vi "64 RMS.vi"() -> ()   [LabVIEW 2017]
uses:
  <vilib>/Analysis/baseanly.llb/Mean (DBL).vi
  <vilib>/Analysis/NI_AALBase.lvlib
panel:
  out "TDC 32 Width":dbl[](graph)=[-0.6783163457252961, 34.80339865309444, -9.301868316936371, -18.575029046661424, -30.46824115548442, -36.068889974290876, -48.12167844719457, -62.45045124910451, -82.61219931936799, -67.52504545488544, -82.18213797919361, -74.58060582693615, -82.56997925436134, -51.89278804838313, -74.89460611630447, -18.140506580336282, -54.34241861431395, 120.78238637788458, 104.77997514317252, 69.37552504098075, 102.67355117145733, 61.80624599007051, 69.19828291963655, 56.38383575637289, 65.54038193174377, 81.65259235989721, 59.02039418272081, 52.81620434909051, 72.46570862393186, 17.962024313646307, 60.3235058067138, 51.75675031672855, 56.5848106452265, 45.431151381143735, 48.336679201226005, 10.391614557583782, 32.39305706018139, -12.86505630083905, -24.22287886989784, -15.211095332141797, -12.471040103140627, -7.020617140658874, -16.741559776427525, -21.080385174466098, -1.214389654830226, -36.76592185679817, -45.26070308895697, 15.57295580171187, -33.053175507633306, -37.140407160289904, -62.42416008241627, -12103.8678050851, -12121.48251904026, -12111.404616944672, -12129.543609930342, -12139.843547353412, -12129.977664947211, -12131.654983175655, -12134.08824321654, -12113.99974215647, -12112.278518000594, -12102.802796490787, -12126.243066943878]
  in  "PMT Num Channel":i32=64
  out "TDC 32 Pre RMS 2":dbl[](graph)
  out "TDC 32 Mean 2":dbl[](graph)=[0.0, -135.09479077989525, -421.8271505306632, -840.8446778298572, -1162.0976991710277, -1612.7332666304121, -2198.59017285921, -2560.663067796938, -2635.055025403253, -2231.1708563380016, -2195.002950279124, -1580.3730444661662, -1326.1414516725524, -1107.6882588350188, -612.4428634104521, -418.3344995069555, -181.55837998871735, -553.1504945996667, -839.4835673473254, -924.4151651207177, -1354.6877899459462, -1876.633411331489, -2226.4242092546738, -2150.03492136841, -1877.2355072689136, -1778.347255928683, -1323.9390592383058, -710.8504740240475, -576.8078492540101, -276.2199801150382, 188.3439838906523, 324.0294182912872]
  in  "Width大于信号周期":dbl=10000.0
  in  "Width小于信号周期":dbl=10000000.0
  in  "Post大于信号周期":dbl
  in  "Post小于信号周期":dbl=25000.0
  in  "Pre大于信号周期":dbl
  in  "Pre小于信号周期":dbl=25500.0
  in  "min bin 3":i32=30
  in  "length 3":dbl=60.0 format="%#_13g"
  out "Fitting RMS 2":dbl=7.681145747868608
  out "Array 3":dbl[](array[numeric])=[0.0, 4.475261371081126, 3.162544268461357, 2.924189728577925, 4.462904629576637, 4.688451182126854, 4.149795436251731, 5.294255584605741, 4.358239562408714, 5.964552050869855, 6.274622613679179, 4.820259051506523, 6.210237569711836, 6.202576111524344, 5.12191356026047, 5.902693786358635, 7.264783281499365, 3.8782644204457255, 6.15892371349985, 5.6565100281603495, 5.6445556358933535, 5.586306730858833, 5.237143591840878, 7.583770998832869, 5.692958951594319, 4.962442273104816, 5.385209825663387, 6.281457453209248, 4.513090750771602, 4.263987705812667, 4.44121495773946, 4.025581062368119]
  out "index 3":i32
  out "Fitting RMS":dbl=3.2734913936560712
  in  "String":string
  out "cal 3":cluster{"cal 2":dbl[]}[](graph)=[{"cal 2"=[0.0, 4.114652313560727, 4.4615536591768565, 4.487541869293653, 4.305805863389491, 4.3919731471213845, 4.293945065128187, 3.9563450305643455, 4.781590920128164, 4.566725321246964, 3.769905678360813, 3.996457081541512, 3.6292687673693096, 4.6661813542211945, 3.9547291663385615, 4.0878496237189195, 5.193601946935443, 4.363571307074085, 4.620812080547306, 4.68636099579301, 4.522595786195377, 4.94953151612554, 4.20504962269455, 4.5858390402275155, 4.63399159695198, 5.369311213376012, 4.839189336674422, 5.220406472025208, 4.474735648398492, 4.088850343918244, 5.168763522181636, 6.520882565694521]}, {"cal 2"=[0.0, 4.475261371081126, 3.162544268461357, 2.924189728577925, 4.462904629576637, 4.688451182126854, 4.149795436251731, 5.294255584605741, 4.358239562408714, 5.964552050869855, 6.274622613679179, 4.820259051506523, 6.210237569711836, 6.202576111524344, 5.12191356026047, 5.902693786358635, 7.264783281499365, 3.8782644204457255, 6.15892371349985, 5.6565100281603495, 5.6445556358933535, 5.586306730858833, 5.237143591840878, 7.583770998832869, 5.692958951594319, 4.962442273104816, 5.385209825663387, 6.281457453209248, 4.513090750771602, 4.263987705812667, 4.44121495773946, 4.025581062368119]}]
  out "post mean":dbl=3.154553539854668 format="%0.2f"
  out "pre mean":dbl=2.9457244798960076 format="%0.2f"
  out "mean":dbl=3.050139009875338 format="%0.2f"
  out "TDC 32 Mean":dbl[](graph)=[0.0, -36.996434242557854, -31.313627065973662, -21.077383139604187, 2.6241265645144156, 24.179747631180753, 2.7343041360305027, -30.431283162442877, 18.929146350224407, 35.626740082844826, 54.916933857204114, 38.31421986338976, 51.65477997851549, 14.6334264613231, 63.72841817768095, 23.989321006770542, 66.44079691895976, -2.810644526473722, -130.76823833968274, -83.04624565073621, -125.70406933559532, -120.26787383317914, -78.81175803979941, -76.26600047186471, -124.72740831159858, -86.923123129569, -112.60533075805586, -80.56440015739442, -93.43063512184393, -101.85614274031633, -58.36081718509212, -71.76328499120083, -110.40069925774178, -83.1465185905702, -45.32711285598063, -52.80271804532156, -12.349259962253637, -6.78472000965643, 19.69497358721831, -2.6869885934701703, -0.49182237994686606, 30.518656522275663, 22.293804071974055, 12.59663288956947, 6.842670087488456, -17.05003568301032, -5.350597835875373, 17.811916976727968, 3.882015796675974, 36.65946347529074, 6.0177148567894845, 50.32927610106109, 12120.695864120817, 12102.81226011086, 12106.473027754682, 12166.901296162248, 12132.2829669936, 12127.91935865152, 12112.96936554167, 12147.343894796079, 12110.6243252432, 12131.056590850796, 12139.238157468637, 12131.590924217124]
  out "cal 2":cluster{"cal 2":dbl[]}[](graph)=[{"cal 2"=[0.0, 2.7660591431756636, 2.7965204008011693, 2.8371751476759077, 2.9687865748397413, 2.586901217982678, 3.049603258650606, 2.7769429000377315, 2.84337439739946, 2.8079919817042938, 3.0911315648646758, 3.2064489186545337, 2.899310886145602, 3.307008327270206, 2.90831028930621, 3.418607736993944, 2.991778379065165, 3.1044560328618847, 2.8635383951772084, 2.874130589680789, 2.9022368004793555, 3.163327380796549, 3.095057673087491, 3.017902652759673, 2.576954383186888, 2.830253201212209, 3.0679451279799497, 3.0082959014666697, 3.0310317195983947, 3.086400717933539, 3.148829226197087, 2.9710914995519375, 3.1027831871783977, 3.081309500479302, 3.0130135668078113, 3.129637095585219, 3.027166346566586, 2.9275365165118745, 2.856538471442075, 2.802569477786886, 3.0221181838965676, 3.0701711249384998, 3.123228137730836, 3.091689538434885, 2.9169499835656345, 3.2171659335383005, 2.9161334166545054, 3.156954195781715, 3.4267992870209865, 2.763287658090245, 2.9777255480248073, 2.9171925704161987, 2.966870830785901, 2.8776645339995643, 2.60596569982052, 3.0716380760397723, 3.017306157019706, 3.004246243333819, 3.0730206629174335, 3.037578499717302, 3.078007168642431, 2.952557438808163, 3.1355522957812796, 3.168586939490012]}, {"cal 2"=[0.0, 2.8996020427561886, 2.9895727123516944, 3.063090569150334, 2.885454310411448, 3.308199160492238, 2.8929806886235356, 3.1201842138819305, 2.7175292754088933, 3.2853680454446224, 3.4020354438142792, 3.4286914898543315, 3.276135144500932, 3.36085761963916, 3.2767937308862245, 3.4073773280141952, 3.2097845553822832, 3.124423833048686, 3.1124194853662472, 3.201558278093965, 3.025530124534342, 2.9839245800581313, 3.1800101711476065, 2.955793860682045, 3.2429221091245233, 2.9937445582570916, 2.9432208257186643, 3.149619864411783, 3.2718821210784856, 3.5334178494461552, 3.4373358702503625, 3.3677472097516246, 3.6041042638956777, 3.4388784451735224, 3.4801093500010754, 3.046059251257246, 3.2320592552775222, 3.193104588644505, 3.352133295854613, 3.5929937145986566, 3.1733456599894576, 3.1702333717532403, 3.1843260581136894, 3.1915311308326313, 2.990203209342016, 3.111223016994537, 3.2063459292445002, 3.3140730928092825, 3.406148065853031, 3.46159765385004, 3.3981654931647975, 3.162194273391769, 3.275580228314425, 3.1277255614951605, 3.0185159184215657, 3.078378013806016, 3.0340271987123693, 3.172771154107615, 3.4402058505393294, 3.1092898332858816, 3.2674772912638206, 3.1359517649189352, 3.201976150553741, 3.2734913936560712]}]
  in  "min bin 2":i32=30
  in  "length 2":dbl=60.0 format="%#_13g"
  out "Array 2":dbl[](array[numeric])=[0.0, 2.8996020427561886, 2.9895727123516944, 3.063090569150334, 2.885454310411448, 3.308199160492238, 2.8929806886235356, 3.1201842138819305, 2.7175292754088933, 3.2853680454446224, 3.4020354438142792, 3.4286914898543315, 3.276135144500932, 3.36085761963916, 3.2767937308862245, 3.4073773280141952, 3.2097845553822832, 3.124423833048686, 3.1124194853662472, 3.201558278093965, 3.025530124534342, 2.9839245800581313, 3.1800101711476065, 2.955793860682045, 3.2429221091245233, 2.9937445582570916, 2.9432208257186643, 3.149619864411783, 3.2718821210784856, 3.5334178494461552, 3.4373358702503625, 3.3677472097516246, 3.6041042638956777, 3.4388784451735224, 3.4801093500010754, 3.046059251257246, 3.2320592552775222, 3.193104588644505, 3.352133295854613, 3.5929937145986566, 3.1733456599894576, 3.1702333717532403, 3.1843260581136894, 3.1915311308326313, 2.990203209342016, 3.111223016994537, 3.2063459292445002, 3.3140730928092825, 3.406148065853031, 3.46159765385004, 3.3981654931647975, 3.162194273391769, 3.275580228314425, 3.1277255614951605, 3.0185159184215657, 3.078378013806016, 3.0340271987123693, 3.172771154107615, 3.4402058505393294, 3.1092898332858816, 3.2674772912638206, 3.1359517649189352, 3.201976150553741, 3.2734913936560712]
  out "TOT":dbl[](graph)=[0.0, 2.8996020427561886, 2.9895727123516944, 3.063090569150334, 2.885454310411448, 3.308199160492238, 2.8929806886235356, 3.1201842138819305, 2.7175292754088933, 3.2853680454446224, 3.4020354438142792, 3.4286914898543315, 3.276135144500932, 3.36085761963916, 3.2767937308862245, 3.4073773280141952, 3.2097845553822832, 3.124423833048686, 3.1124194853662472, 3.201558278093965, 3.025530124534342, 2.9839245800581313, 3.1800101711476065, 2.955793860682045, 3.2429221091245233, 2.9937445582570916, 2.9432208257186643, 3.149619864411783, 3.2718821210784856, 3.5334178494461552, 3.4373358702503625, 3.3677472097516246, 3.6041042638956777, 3.4388784451735224, 3.4801093500010754, 3.046059251257246, 3.2320592552775222, 3.193104588644505, 3.352133295854613, 3.5929937145986566, 3.1733456599894576, 3.1702333717532403, 3.1843260581136894, 3.1915311308326313, 2.990203209342016, 3.111223016994537, 3.2063459292445002, 3.3140730928092825, 3.406148065853031, 3.46159765385004, 3.3981654931647975, 3.162194273391769, 3.275580228314425, 3.1277255614951605, 3.0185159184215657, 3.078378013806016, 3.0340271987123693, 3.172771154107615, 3.4402058505393294, 3.1092898332858816, 3.2674772912638206, 3.1359517649189352, 3.201976150553741, 3.2734913936560712]
  out "index 2":i32=126
  in  "length":dbl=200.0 format="%#_13g"
  in  "min bin":i32=100
  out "index":i32=126
  out "TOA":dbl[](graph)=[0.0, 2.7660591431756636, 2.7965204008011693, 2.8371751476759077, 2.9687865748397413, 2.586901217982678, 3.049603258650606, 2.7769429000377315, 2.84337439739946, 2.8079919817042938, 3.0911315648646758, 3.2064489186545337, 2.899310886145602, 3.307008327270206, 2.90831028930621, 3.418607736993944, 2.991778379065165, 3.1044560328618847, 2.8635383951772084, 2.874130589680789, 2.9022368004793555, 3.163327380796549, 3.095057673087491, 3.017902652759673, 2.576954383186888, 2.830253201212209, 3.0679451279799497, 3.0082959014666697, 3.0310317195983947, 3.086400717933539, 3.148829226197087, 2.9710914995519375, 3.1027831871783977, 3.081309500479302, 3.0130135668078113, 3.129637095585219, 3.027166346566586, 2.9275365165118745, 2.856538471442075, 2.802569477786886, 3.0221181838965676, 3.0701711249384998, 3.123228137730836, 3.091689538434885, 2.9169499835656345, 3.2171659335383005, 2.9161334166545054, 3.156954195781715, 3.4267992870209865, 2.763287658090245, 2.9777255480248073, 2.9171925704161987, 2.966870830785901, 2.8776645339995643, 2.60596569982052, 3.0716380760397723, 3.017306157019706, 3.004246243333819, 3.0730206629174335, 3.037578499717302, 3.078007168642431, 2.952557438808163, 3.1355522957812796, 3.168586939490012]
  out "Array":dbl[](array[numeric])=[0.0, 2.7660591431756636, 2.7965204008011693, 2.8371751476759077, 2.9687865748397413, 2.586901217982678, 3.049603258650606, 2.7769429000377315, 2.84337439739946, 2.8079919817042938, 3.0911315648646758, 3.2064489186545337, 2.899310886145602, 3.307008327270206, 2.90831028930621, 3.418607736993944, 2.991778379065165, 3.1044560328618847, 2.8635383951772084, 2.874130589680789, 2.9022368004793555, 3.163327380796549, 3.095057673087491, 3.017902652759673, 2.576954383186888, 2.830253201212209, 3.0679451279799497, 3.0082959014666697, 3.0310317195983947, 3.086400717933539, 3.148829226197087, 2.9710914995519375, 3.1027831871783977, 3.081309500479302, 3.0130135668078113, 3.129637095585219, 3.027166346566586, 2.9275365165118745, 2.856538471442075, 2.802569477786886, 3.0221181838965676, 3.0701711249384998, 3.123228137730836, 3.091689538434885, 2.9169499835656345, 3.2171659335383005, 2.9161334166545054, 3.156954195781715, 3.4267992870209865, 2.763287658090245, 2.9777255480248073, 2.9171925704161987, 2.966870830785901, 2.8776645339995643, 2.60596569982052, 3.0716380760397723, 3.017306157019706, 3.004246243333819, 3.0730206629174335, 3.037578499717302, 3.078007168642431, 2.952557438808163, 3.1355522957812796, 3.168586939490012]
  in  "base channel":i32
  in  "file path (dialog if empty)":path=path "G:/tdc/2017/data/test_20250326_071915.csv"
  # "G:\\tdc\\2017\\test_20230328_085653.csv"
  # "G:\\tdc\\2017\\test_20230905_020448.csv   2.8 ps"
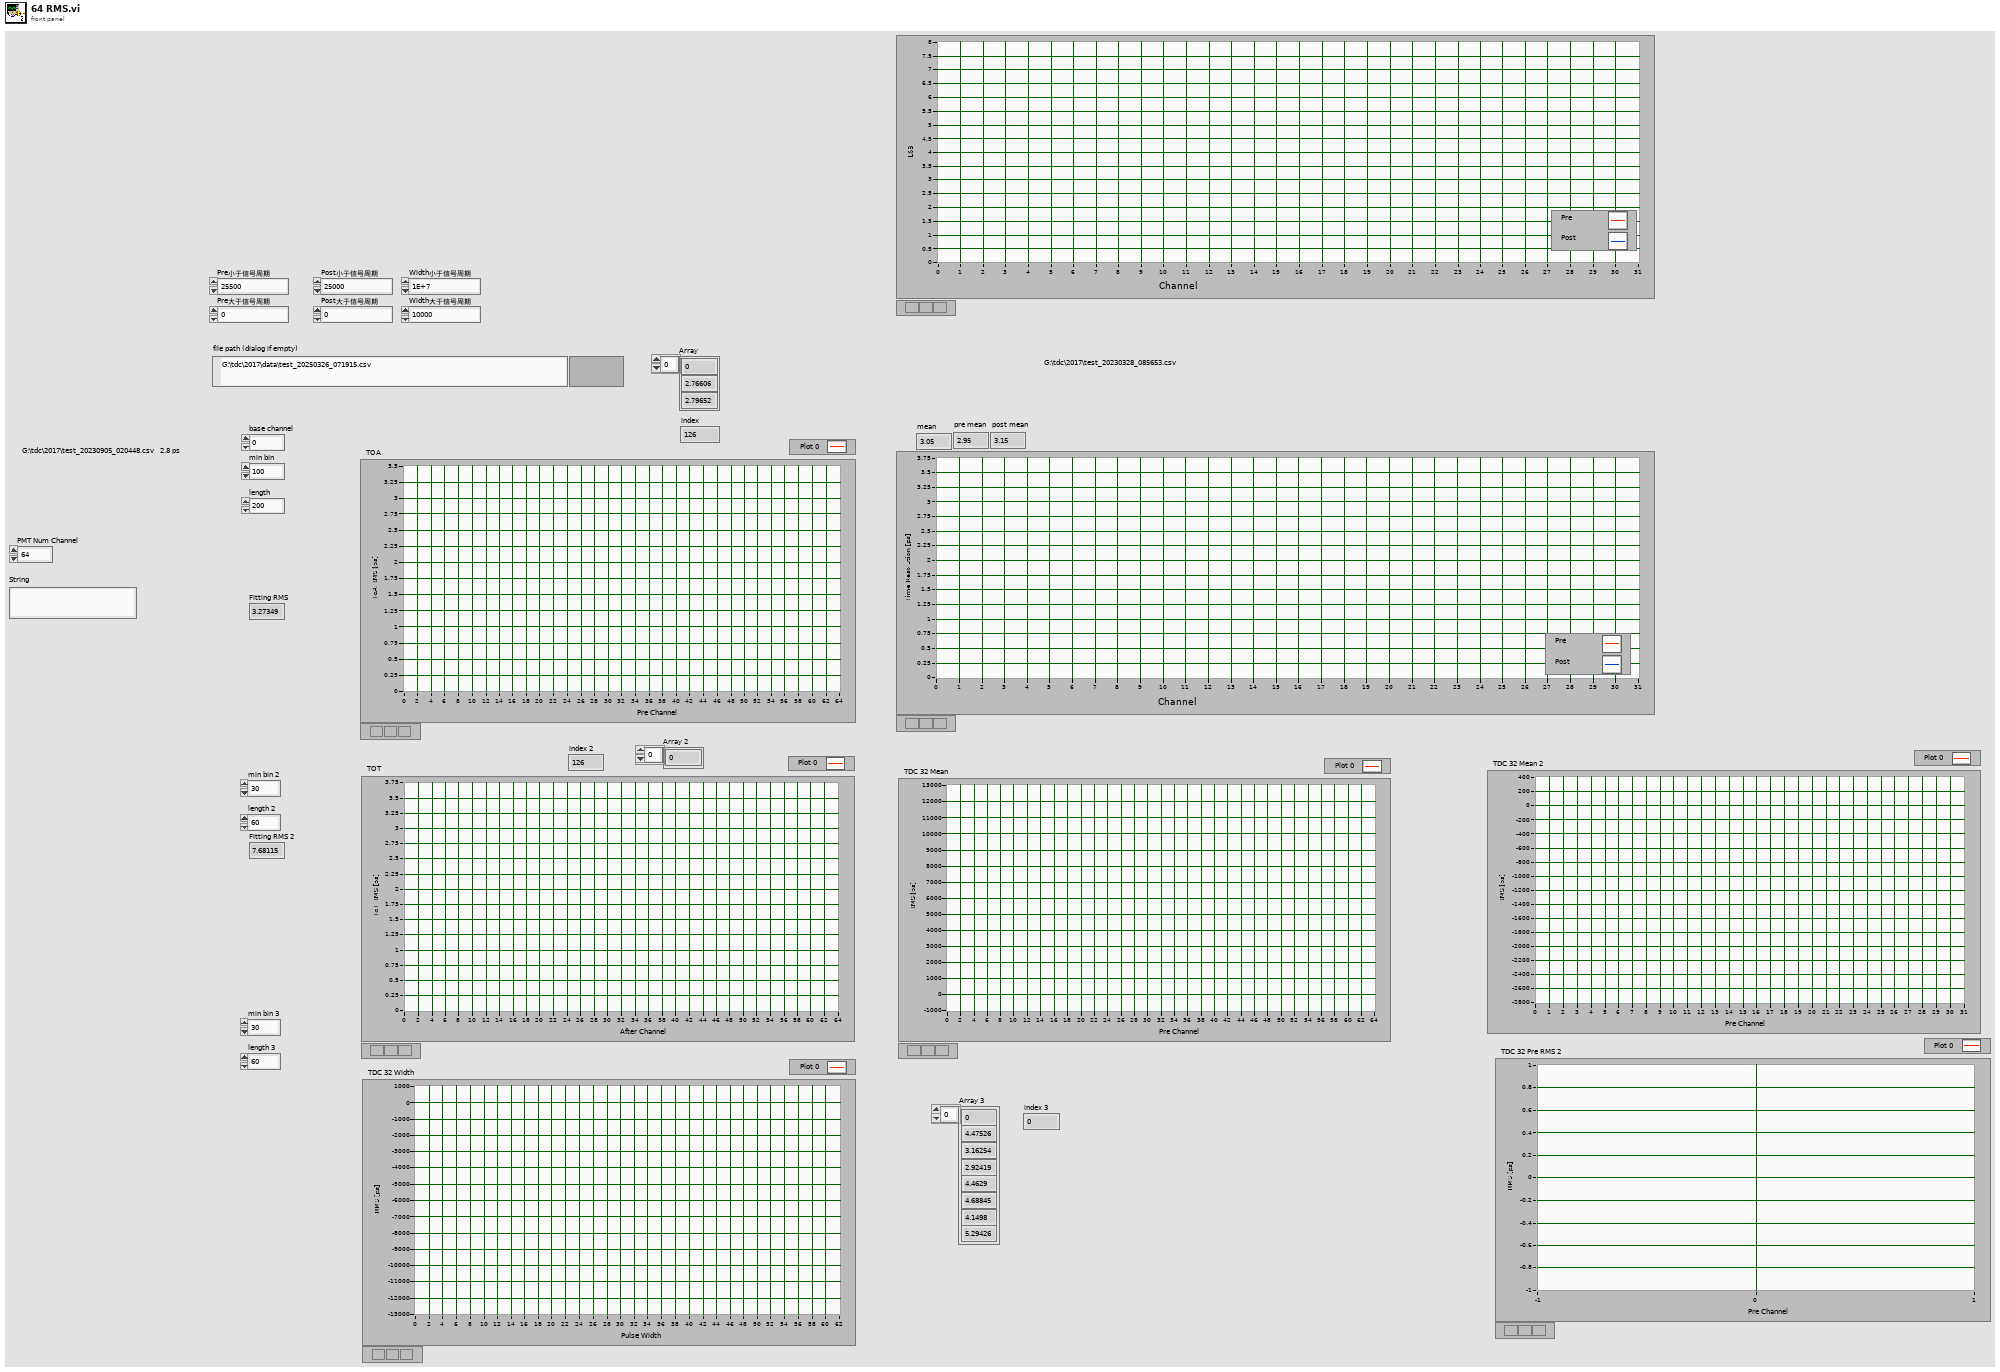
[diagram p1: front panel]
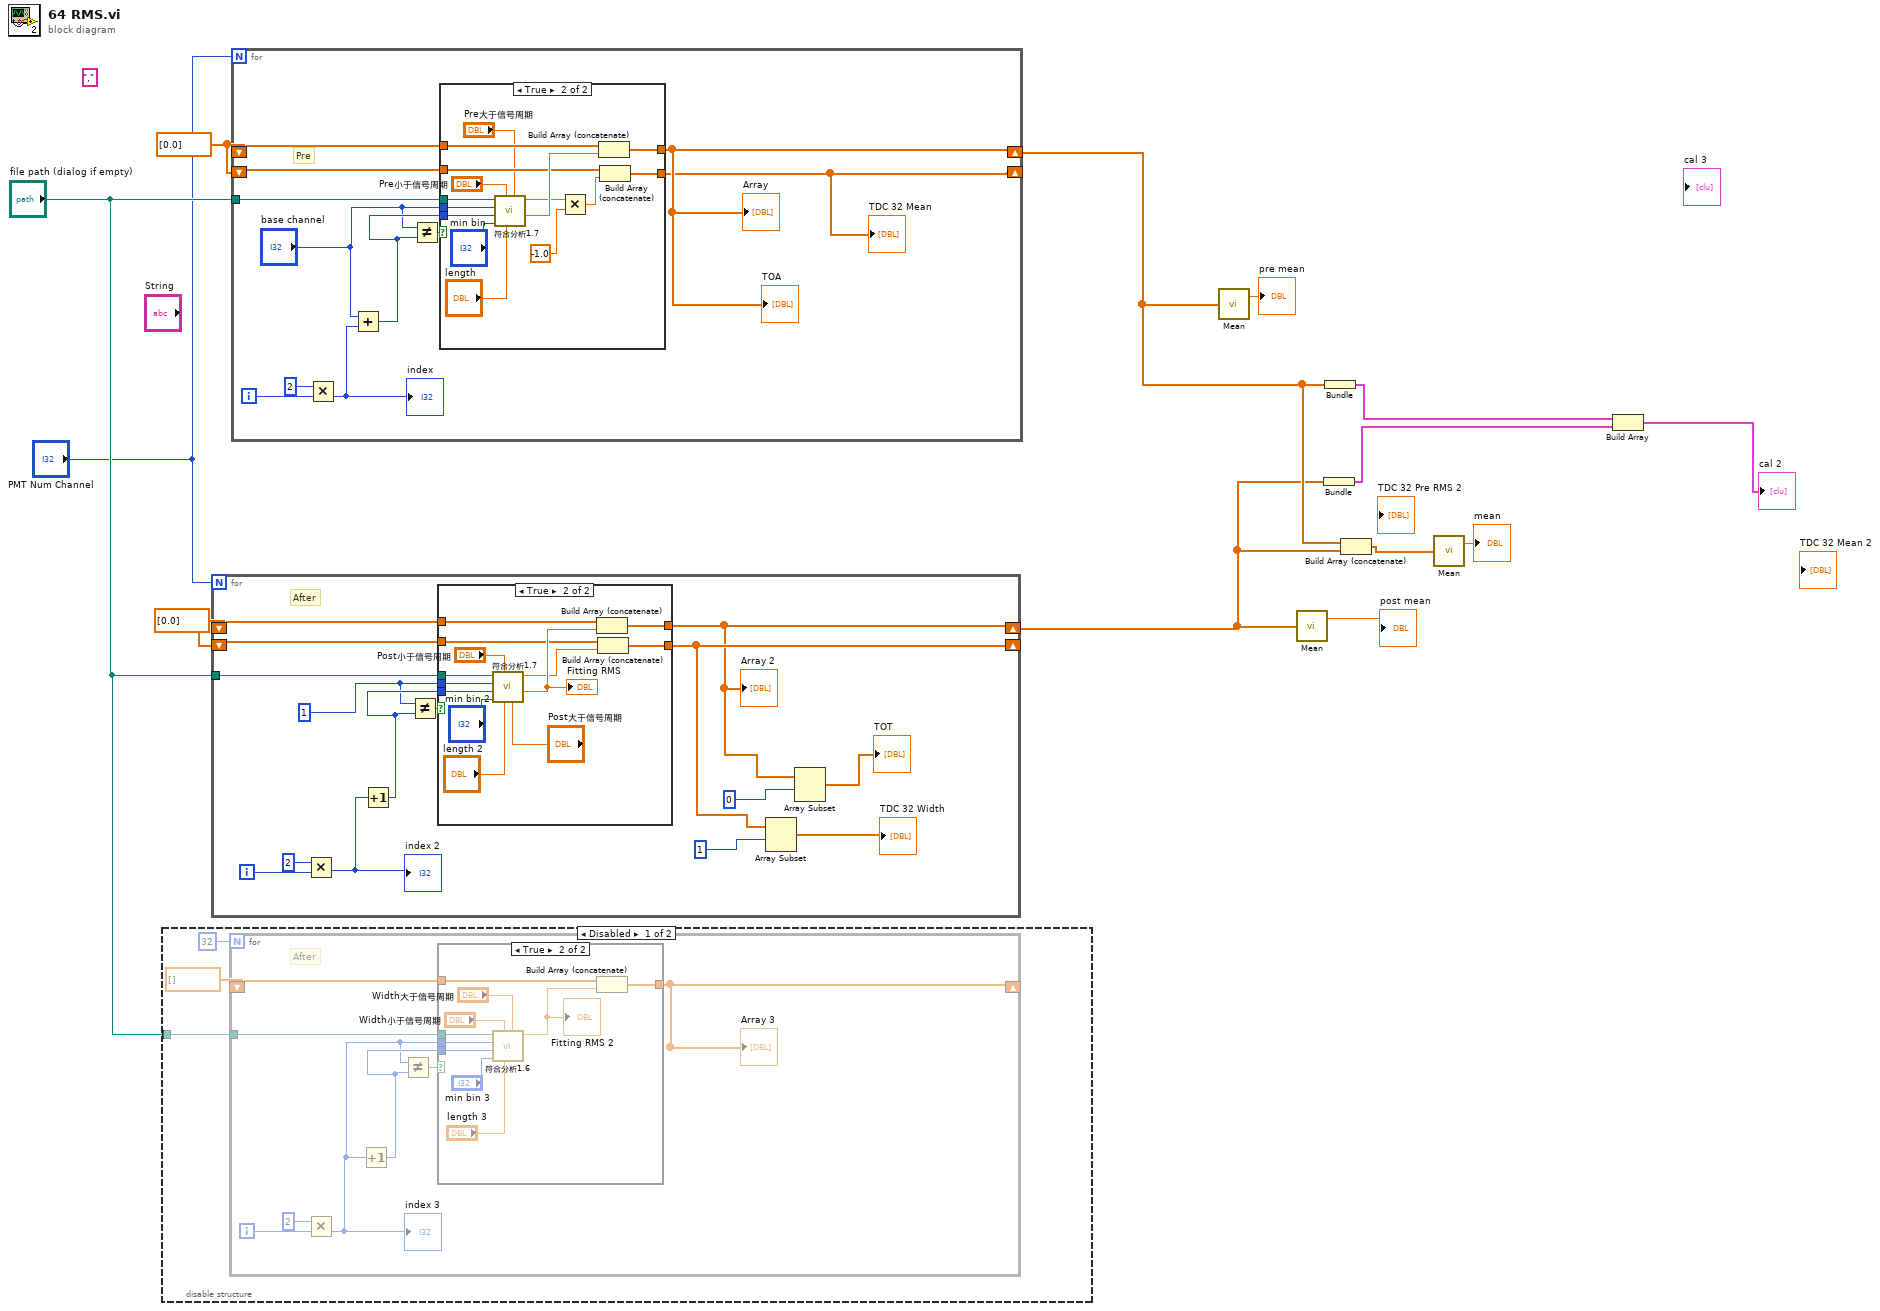
[diagram p0: block diagram]
diagram:
  w1 = dbl[] [0.0]
  (unwired) "," ("delimiter (\\t)")
  w10 = dbl[] [0.0]
  n1 = disable-structure shown="Disabled" {
    disable-tunnel: "file path (dialog if empty)" -> [w14 _]
    frame Disabled {
      n2 = for {
        N: 32 -> [_]
        tunnel: w14 -> [w24]
        shift-right: [w20] -> _
        shift-left: dbl[] [] -> [w21]
        i -> [w22]
        # "After"
        n3 = Multiply(x=2, y=w22) -> (x*y=w17:i32)
        "index 3" <- w17
        n4 = Increment(x=w17) -> (x+1=w18:i32)
        n5 = Not Equal?(x=w17, y=w18) -> (x != y?=w23:bool)
        n6 = case shown="True" w23 {
          tunnel: w24 -> [_ w35]
          tunnel: w17 -> [_ w34]
          tunnel: w18 -> [_ w33]
          tunnel: [w25 w32] -> w20
          tunnel: w21 -> [w25 w31]
          frame False {
          }
          frame True {
            n7 = call "符合分析1.6.vi"("大于信号周期"="Width大于信号周期", "length"="length 3", "小于信号周期"="Width小于信号周期", "min bin"="min bin 3", "通道B"=w33, "通道A"=w34, "file path (dialog if empty)"=w35) -> ("mean[ps]"=w28:dbl)  [unwired: 4 out]
            "Fitting RMS 2" <- w28
            n8 = Build Array (concatenate)(w31, w28) -> (w32:dbl[])
          }
        }
        "Array 3" <- w20
      }
    }
    frame Enabled {
    }
  }
  n9 = for {
    N: "PMT Num Channel" -> [_]
    tunnel: "file path (dialog if empty)" -> [w50]
    shift-right: [w39] -> w8
    shift-left: w1 -> [w47]
    shift-right: [w43] -> _
    shift-left: w1 -> [w44]
    i -> [w48]
    w37 = 1 ("x")
    # "After"
    n10 = Multiply(x=2, y=w48) -> (x*y=w36:i32)
    "index 2" <- w36
    n11 = Increment(x=w36) -> (x+1=w45:i32)
    n12 = Not Equal?(x=w37, y=w45) -> (x != y?=w49:bool)
    n13 = case shown="True" w49 {
      tunnel: w50 -> [_ w65]
      tunnel: w37 -> [_ w64]
      tunnel: w45 -> [_ w63]
      tunnel: [w52 w62] -> w39
      tunnel: w47 -> [w52 w61]
      tunnel: w44 -> [w51 w55]
      tunnel: [w51 w53] -> w43
      frame False {
      }
      frame True {
        n14 = call "符合分析1.7.vi"("大于信号周期"="Post大于信号周期", "length"="length 2", "小于信号周期"="Post小于信号周期", "min bin"="min bin 2", "通道B"=w63, "通道A"=w64, "file path (dialog if empty)"=w65) -> ("Fitting Sigma"=w60:dbl, "mean[ps]"=w54:dbl)  [unwired: 1 in, 2 out]
        "Fitting RMS" <- w60
        n15 = Build Array (concatenate)(w61, w60) -> (w62:dbl[])
        n16 = Build Array (concatenate)(w55, w54) -> (w53:dbl[])
      }
    }
    "Array 2" <- w39
    n17 = Array Subset(array=w43, index=1) -> (→"TDC 32 Width":dbl[])  [unwired: 1 in]
    n18 = Array Subset(array=w39, index=0) -> (→"TOT":dbl[])  [unwired: 1 in]
  }
  n19 = for {
    N: "PMT Num Channel" -> [_]
    tunnel: "file path (dialog if empty)" -> [w76]
    shift-right: [w72] -> w9
    shift-left: w10 -> [w73]
    shift-right: [w66] -> _
    shift-left: w10 -> [w67]
    i -> [w74]
    # "Pre"
    n20 = Multiply(x=2, y=w74) -> (x*y=w71:i32)
    "index" <- w71
    n21 = Add(x="base channel", y=w71) -> (x+y=w69:i32)
    n22 = Not Equal?(x="base channel", y=w69) -> (x != y?=w75:bool)
    n23 = case shown="True" w75 {
      tunnel: w76 -> [_ w93]
      tunnel: "base channel" -> [_ w92]
      tunnel: w69 -> [_ w91]
      tunnel: [w78 w90] -> w72
      tunnel: w73 -> [w78 w89]
      tunnel: w67 -> [w77 w85]
      tunnel: [w77 w84] -> w66
      frame False {
      }
      frame True {
        n24 = call "符合分析1.7.vi"("大于信号周期"="Pre大于信号周期", "length"="length", "小于信号周期"="Pre小于信号周期", "min bin"="min bin", "通道B"=w91, "通道A"=w92, "file path (dialog if empty)"=w93) -> ("Fitting Sigma"=w88:dbl, "mean[ps]"=w80:dbl)  [unwired: 1 in, 2 out]
        n25 = Multiply(x=w80, y=-1.0) -> (x*y=w81:dbl)
        n26 = Build Array (concatenate)(w89, w88) -> (w90:dbl[])
        n27 = Build Array (concatenate)(w85, w81) -> (w84:dbl[])
      }
    }
    "Array" <- w72
    "TOA" <- w72
    "TDC 32 Mean" <- w66
  }
  n28 = call-poly <vilib>:"Mean.vi"("X"=w9) -> ("mean"=→"pre mean":dbl)  [unwired: 1 out]
  n29 = call-poly <vilib>:"Mean.vi"("X"=w8) -> ("mean"=→"post mean":dbl)  [unwired: 1 out]
  n30 = Bundle(w8) -> (w13:cluster{dbl[]})  [unwired: 1 in]
  n31 = Bundle(w9) -> (w11:cluster{dbl[]})  [unwired: 1 in]
  n32 = Build Array (concatenate)(w9, w8) -> (w7:dbl[])
  n33 = call-poly <vilib>:"Mean.vi"("X"=w7) -> ("mean"=→"mean":dbl)  [unwired: 1 out]
  n34 = Build Array(w11, w13) -> (→"cal 2":cluster{dbl[]}[])
